vi "Configure Basic Jitter.vi"(0 "VISA resource name":refnum<visa-resource-name>, 1 "Jitter Analysis Gain (0: jg1x)":i32(ring) items=["jg1x", "jg10x", "jg20x", "jg30x"], 2 "Invert EQ (T: Enable)":bool=TRUE, 5 "Analyzer (0: A0)":i32(ring) items=["A0", "A1"], 7 "Jitter Domain (0: jdTime)":i32(ring) items=["jdTime", "jdFreq"], 9 "Jitter Units (0: muUI)":i32(ring) items=["muUI", "muSec"], 11 "error in (no error)":errorcluster, 12 "Time Weighting Filter (0: adNoWt)":i32(ring) items=["adNoWt", "adAWt", "adCMsg", "adCCITT", "adCCIRwtd", "adCCIRunwtd", "adCCIR2kHz"]) -> (4 "VISA resource name out":refnum<visa-resource-name>, 15 "error out":errorcluster)   [LabVIEW 2014, in "Stanford Research SR1.lvlib"]
doc: "Configures the basic attributes of the Jitter Analyzer."
uses:
  Stanford Research SR1.lvlib
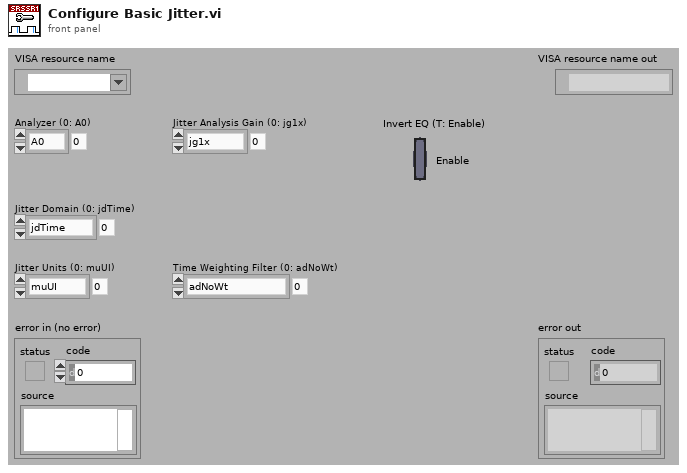
[diagram p1: front panel]
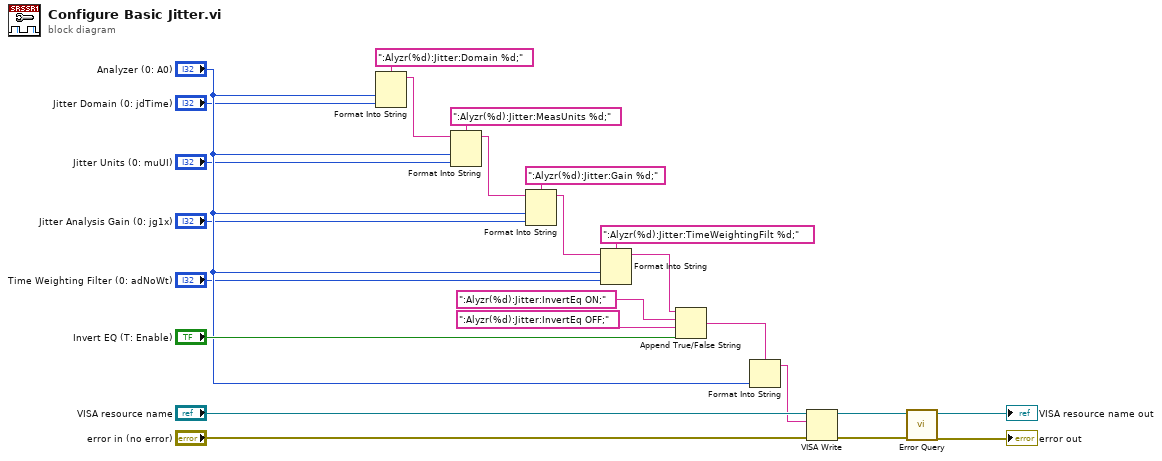
[diagram p0: block diagram]
diagram:
  n1 = Format Into String(format string=":Alyzr(%d):Jitter:Domain %d;", "Analyzer (0: A0)", "Jitter Domain (0: jdTime)") -> (resulting string=w23:string)  [unwired: 2 in, 1 out]
  n2 = Format Into String(format string=":Alyzr(%d):Jitter:MeasUnits %d;", initial string=w23, "Analyzer (0: A0)", "Jitter Units (0: muUI)") -> (resulting string=w21:string)  [unwired: 1 in, 1 out]
  n3 = Format Into String(format string=":Alyzr(%d):Jitter:Gain %d;", initial string=w21, "Analyzer (0: A0)", "Jitter Analysis Gain (0: jg1x)") -> (resulting string=w19:string)  [unwired: 1 in, 1 out]
  n4 = Format Into String(format string=":Alyzr(%d):Jitter:TimeWeightingFilt %d;", initial string=w19, "Analyzer (0: A0)", "Time Weighting Filter (0: adNoWt)") -> (resulting string=w17:string)  [unwired: 1 in, 1 out]
  n5 = Append True/False String(1:"Invert EQ (T: Enable)", 2:":Alyzr(%d):Jitter:InvertEq OFF;", 3:":Alyzr(%d):Jitter:InvertEq ON;", 4:w17) -> (0:w7:string)
  n6 = Format Into String(format string=w7, "Analyzer (0: A0)") -> (resulting string=w6:string)  [unwired: 2 in, 1 out]
  n7 = VISA Write(VISA resource name="VISA resource name", write buffer=w6, error in (no error)="error in (no error)") -> (VISA resource name out=w11:refnum<visa-resource-name>, error out=w10:errorcluster)  [unwired: 1 out]
  n8 = call "Error Query.vi"("error in (no error)"=w10, "VISA resource name"=w11) -> ("error out"=→"error out":errorcluster, "VISA resource name out"=→"VISA resource name out":refnum<visa-resource-name>)  [unwired: 6 in, 2 out]
